vi "ToMotor1CommandSelectFunction.vi"(9 "Encoder 1 count":i64, 10 "theta 0":i32, 11 "theta 1":i32) -> (1 "t":dbl, 2 "Numeric 2":dbl, 3 "Numeric":dbl)   [LabVIEW 2014]
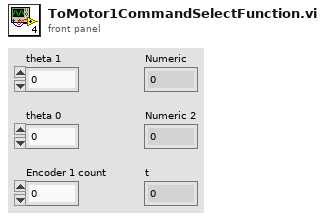
[diagram p1: front panel]
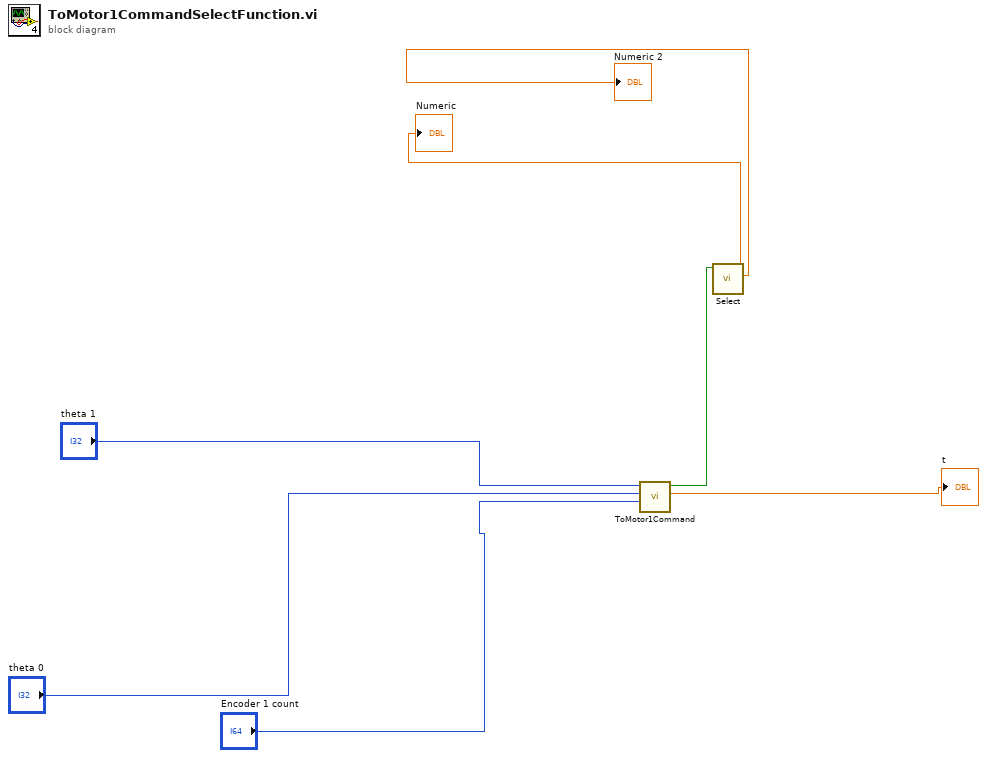
[diagram p0: block diagram]
diagram:
  n1 = call "ToMotor1Command.vi"("Encoder 1 count"="Encoder 1 count", "theta 0"="theta 0", "theta 1"="theta 1") -> ("t"=→"t":dbl, "Boolean"=w6:bool)  [unwired: 7 in]
  n2 = call "Select.vi"("Boolean"=w6) -> ("0th row"=→"Numeric 2":dbl, "1st row"=→"Numeric":dbl)  [unwired: 9 in]
